vi "查询模块.vi"() -> ()   [LabVIEW 2014]
uses:
  <vilib>/addons/database/Connection.llb/Conn ObjectReference.ctl
  <vilib>/addons/database/NI_Database_API.lvlib
panel:
  in  "返回运行界面":bool
  in  "删除选中数据":bool
  in  "保存为其他格式":bool
  in  "本月":bool
  in  "本周":bool
  in  "今天":bool
  in  "昨天":bool
  in  "查询数据显示表格":i32(listbox)
  in  "error out":errorcluster
  in  "连接输出":T1
  in  "Count":string
  in  "查询输入站号":u16(ring) caption="Station" items=["ALL", "10", "20", "30", "40", "50", "60"]
  in  "查询输入模式":u16(ring) caption="Mode" items=["ALL", "46700-D4100(-P/SW)", "46700-D4200(+P/SW)", "46700-D4300(DCT,-P/SW)", "46700-D4400(DCT,+P/SW)"]
  in  "From":string
  in  "To":string
  out "查询指令":string
  in  "OK":bool
  in  "NG":bool
  in  "ALL":bool
  out "查询界面查询条件":u32
  in  "查询输入S/N":string caption="S/N"
  in  "查询界面查询按钮":bool
  # "46700-D4400(DCT,+P/SW):\n                                       Mode:\n                                                      1:46700-D4100(-P/SW)\n                                                      2:46700-D4200(+P/SW)\n                                                      3:46700-D4300(DCT,-P/SW)\n                                                      4:46700-D4400(DCT,+P/SW)\n1506050001                     :\n                                        150605:YY-MM-DD\n                                        0001    :Count"
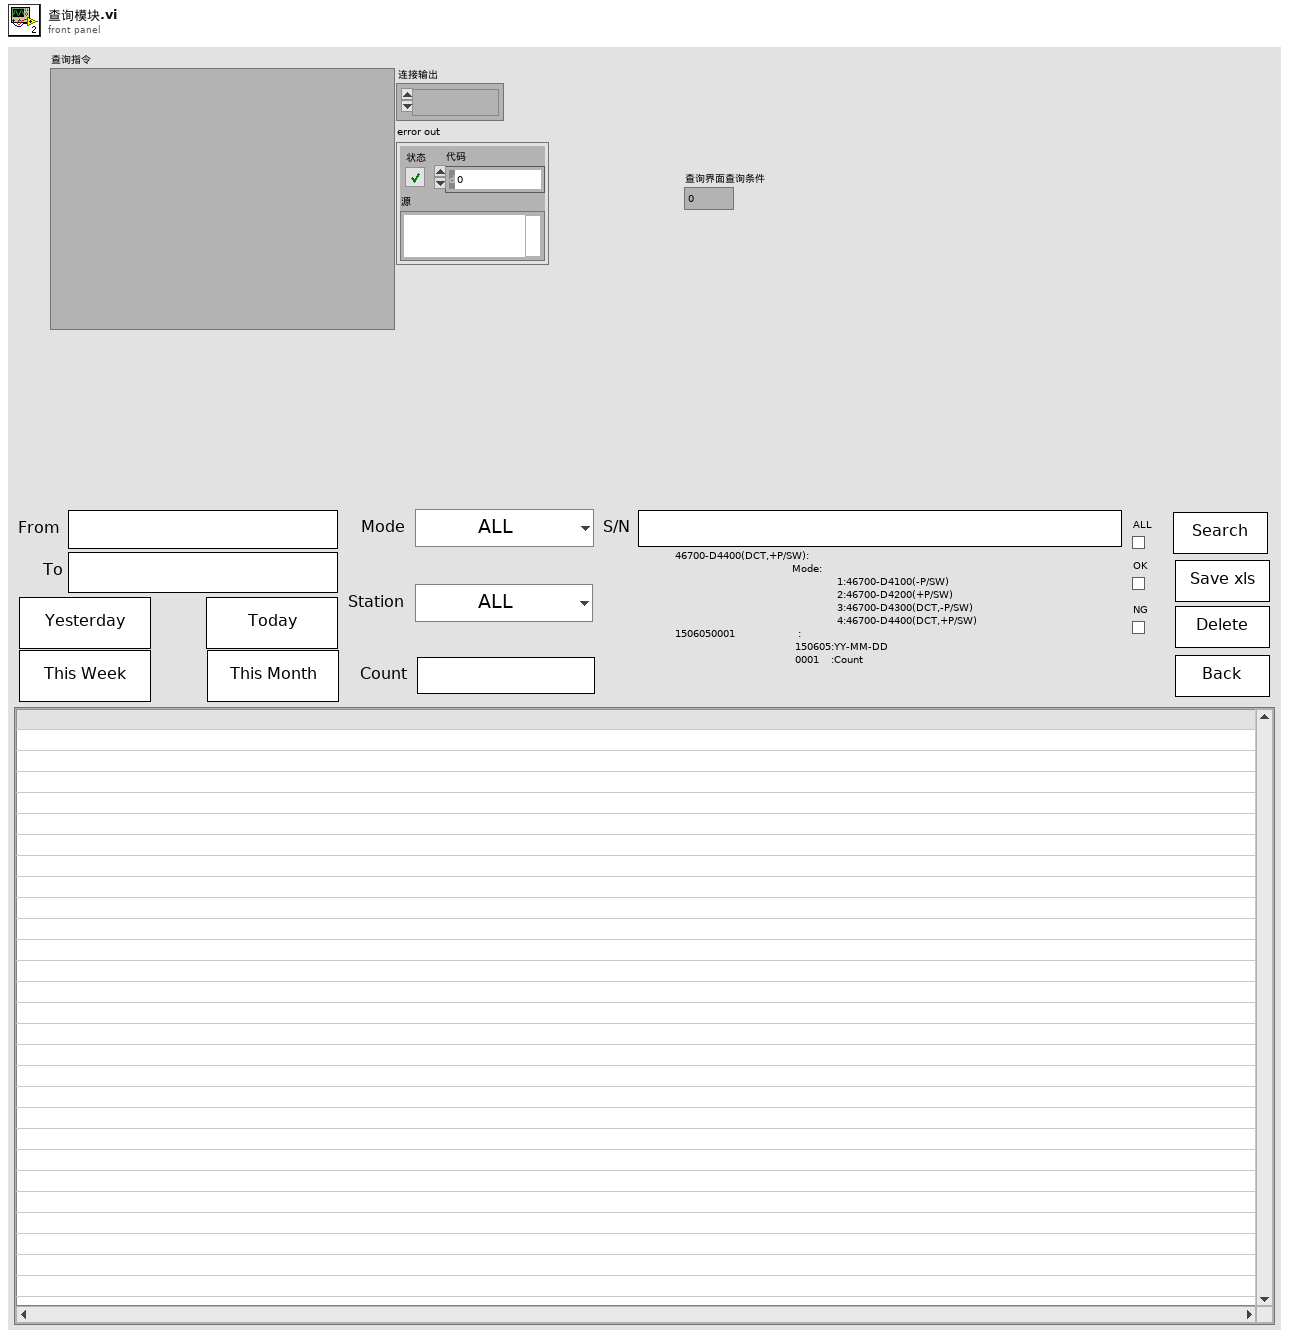
[diagram p1: front panel]
types:
  T1 = typedef "NI_Database_API.lvlib/Conn ObjectReference.ctl" = refnum<k1>
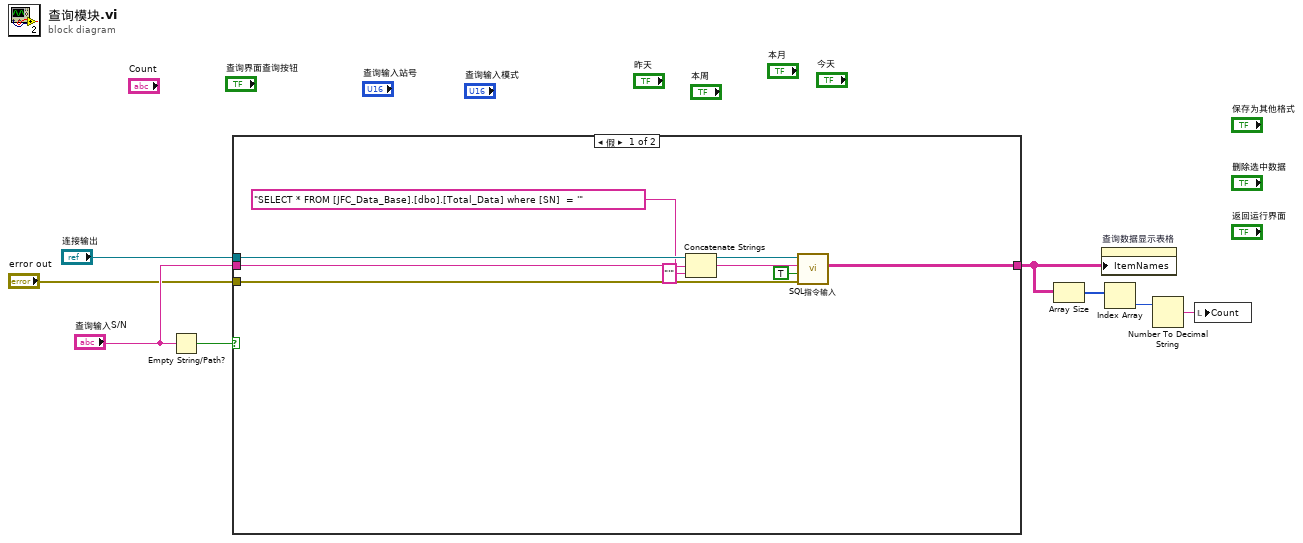
[diagram p0: block diagram]
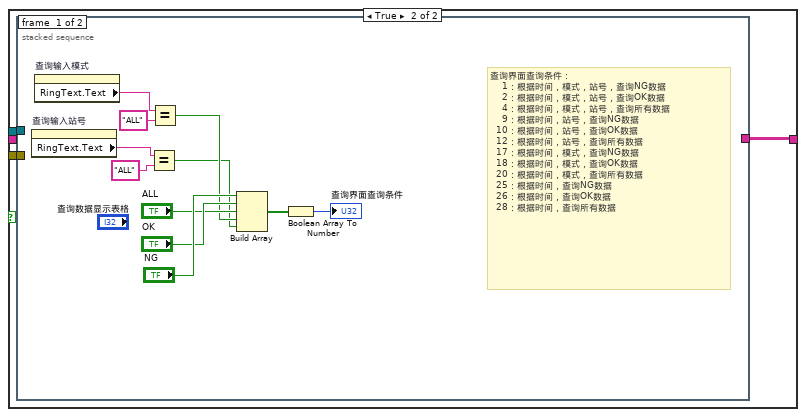
[diagram p2: hidden frame]
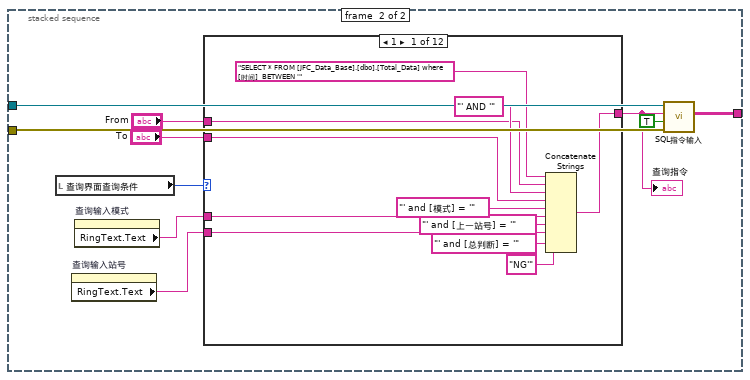
[diagram p3: hidden frame]
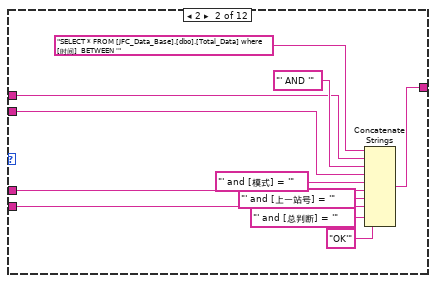
[diagram p4: hidden frame]
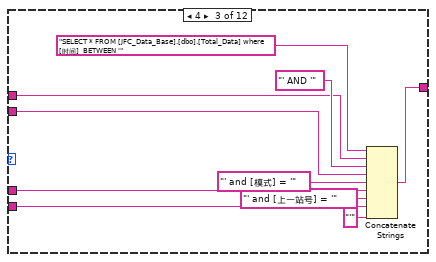
[diagram p5: hidden frame]
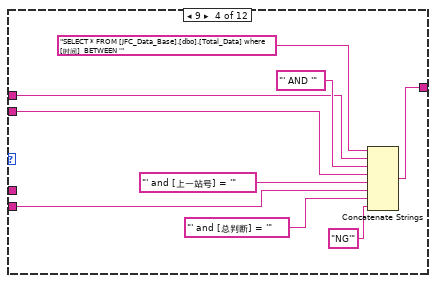
[diagram p6: hidden frame]
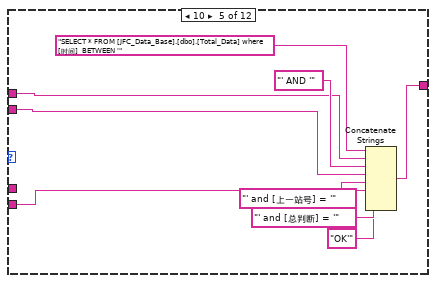
[diagram p7: hidden frame]
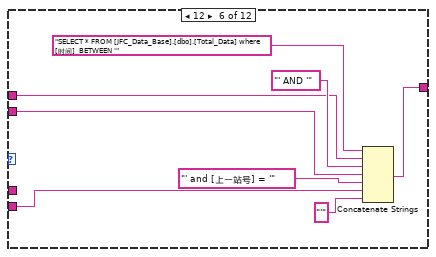
[diagram p8: hidden frame]
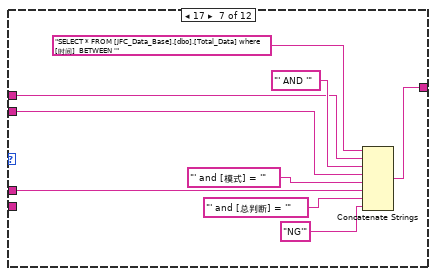
[diagram p9: hidden frame]
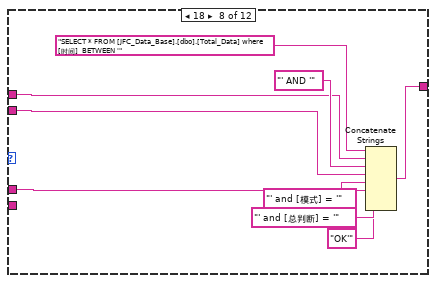
[diagram p10: hidden frame]
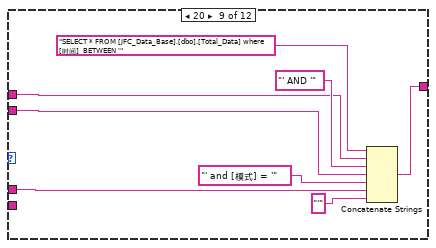
[diagram p11: hidden frame]
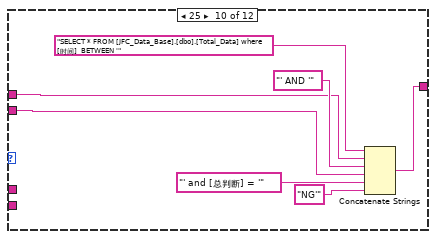
[diagram p12: hidden frame]
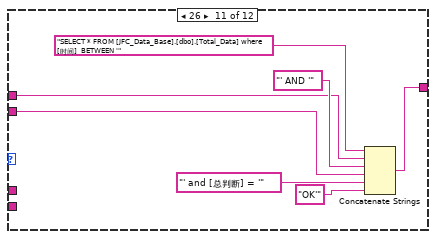
[diagram p13: hidden frame]
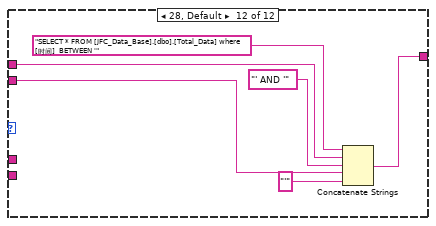
[diagram p14: hidden frame]
diagram:
  n1 = Empty String/Path?(string/path="查询输入S/N") -> (empty?=w8:bool)
  n2 = case shown="假" w8 {
    tunnel: "连接输出" -> [w16 w19]
    tunnel: "error out" -> [w15 w18]
    tunnel: [w13 w17] -> w6
    tunnel: "查询输入S/N" -> [w11 _]
    frame False {
      n3 = Concatenate Strings("SELECT * FROM [JFC_Data_Base].[dbo].[Total_Data] where [SN]  = '" ("SQL query"), w11, "'" ("字符串")) -> (w9:string)
      n4 = call "SQL指令输入.vi"("error in (no error)"=w15, "需要数据？"=TRUE, "SQL query"=w9, "连接输入"=w16) -> ("数据库数据"=w13:string[][])  [unwired: 3 in, 4 out]
    }
    frame True {
      n5 = stacked-sequence {
        tunnel: [_ w40] -> w17
        tunnel: w19 -> [_ w39]
        tunnel: w18 -> [_ w38]
        frame #0 {
          # "查询界面查询条件：\n    1：根据时间，模式，站号，查询NG数据\n    2：根据时间，模式，站号，查询OK数据\n    4：根据时间，模式，站号，查询所有数据\n    9：根据时间，站号，查询NG数据\n  10：根据时间，站号，查询OK数据\n  12：根据时间，站号，查询所有数据\n  17：根据时间，模式，查询NG数据\n  18：根据时间，模式，查询OK数据\n  20：根据时间，模式，查询所有数据\n  25：根据时间，查询NG数据\n  26：根据时间，查询OK数据\n  28：根据时间，查询所有数据"
          n6 = property on="查询输入站号" class="Ring (严格)"() -> ("RingText.Text"=w25:string)  [unwired: 2 in, 2 out]
          n7 = property on="查询输入模式" class="Ring (严格)"() -> ("RingText.Text"=w26:string)  [unwired: 2 in, 2 out]
          n8 = Equal?(x=w25, y="ALL") -> (x = y?=w20:bool)
          n9 = Equal?(x=w26, y="ALL") -> (x = y?=w21:bool)
          n10 = Build Array("NG", "OK", "ALL", w21, w20) -> (w28:bool[])
          n11 = Boolean Array To Number(Boolean array=w28) -> (number=→"查询界面查询条件":u32)
        }
        frame #1 {
          n12 = local read "查询界面查询条件"() -> (w37:u32)
          n13 = property on="查询输入站号" class="Ring (严格)"() -> ("RingText.Text"=w31:string)  [unwired: 2 in, 2 out]
          n14 = property on="查询输入模式" class="Ring (严格)"() -> ("RingText.Text"=w32:string)  [unwired: 2 in, 2 out]
          n15 = case shown="1" w37 {
            tunnel: [w41 w52 w63 w73 w82 w91 w99 w108 w117 w125 w132 w141] -> w36
            tunnel: "From" -> [w49 w56 w67 w76 w85 w95 w102 w111 w120 w127 w134 w140]
            tunnel: "To" -> [w48 w55 w66 w75 w84 w94 w101 w110 w119 w126 w133 w139]
            tunnel: w32 -> [w46 w54 w65 _ _ _ w100 w109 w118 _ _ _]
            tunnel: w31 -> [w44 w53 w64 w74 w83 w93 _ _ _ _ _ _]
            frame 1 {
              n16 = Concatenate Strings("SELECT * FROM [JFC_Data_Base].[dbo].[Total_Data] where [时间]  BETWEEN '" ("SQL query"), w49, "' AND '" ("字符串"), w48, "' and [模式] = '" ("字符串"), w46, "' and [上一站号] = '" ("字符串"), w44, "' and [总判断] = '" ("字符串"), "NG'" ("字符串")) -> (w41:string)
            }
            frame 2 {
              n17 = Concatenate Strings("SELECT * FROM [JFC_Data_Base].[dbo].[Total_Data] where [时间]  BETWEEN '" ("SQL query"), w56, "' AND '" ("字符串"), w55, "' and [模式] = '" ("字符串"), w54, "' and [上一站号] = '" ("字符串"), w53, "' and [总判断] = '" ("字符串"), "OK'" ("字符串")) -> (w52:string)
            }
            frame 4 {
              n18 = Concatenate Strings("SELECT * FROM [JFC_Data_Base].[dbo].[Total_Data] where [时间]  BETWEEN '" ("SQL query"), w67, "' AND '" ("字符串"), w66, "' and [模式] = '" ("字符串"), w65, "' and [上一站号] = '" ("字符串"), w64, "'" ("字符串")) -> (w63:string)
            }
            frame 9 {
              n19 = Concatenate Strings("SELECT * FROM [JFC_Data_Base].[dbo].[Total_Data] where [时间]  BETWEEN '" ("SQL query"), w76, "' AND '" ("字符串"), w75, "' and [上一站号] = '" ("字符串"), w74, "' and [总判断] = '" ("字符串"), "NG'" ("字符串")) -> (w73:string)
            }
            frame 10 {
              n20 = Concatenate Strings("SELECT * FROM [JFC_Data_Base].[dbo].[Total_Data] where [时间]  BETWEEN '" ("SQL query"), w85, "' AND '" ("字符串"), w84, "' and [上一站号] = '" ("字符串"), w83, "' and [总判断] = '" ("字符串"), "OK'" ("字符串")) -> (w82:string)
            }
            frame 12 {
              n21 = Concatenate Strings("SELECT * FROM [JFC_Data_Base].[dbo].[Total_Data] where [时间]  BETWEEN '" ("SQL query"), w95, "' AND '" ("字符串"), w94, "' and [上一站号] = '" ("字符串"), w93, "'" ("字符串")) -> (w91:string)
            }
            frame 17 {
              n22 = Concatenate Strings("SELECT * FROM [JFC_Data_Base].[dbo].[Total_Data] where [时间]  BETWEEN '" ("SQL query"), w102, "' AND '" ("字符串"), w101, "' and [模式] = '" ("字符串"), w100, "' and [总判断] = '" ("字符串"), "NG'" ("字符串")) -> (w99:string)
            }
            frame 18 {
              n23 = Concatenate Strings("SELECT * FROM [JFC_Data_Base].[dbo].[Total_Data] where [时间]  BETWEEN '" ("SQL query"), w111, "' AND '" ("字符串"), w110, "' and [模式] = '" ("字符串"), w109, "' and [总判断] = '" ("字符串"), "OK'" ("字符串")) -> (w108:string)
            }
            frame 20 {
              n24 = Concatenate Strings("SELECT * FROM [JFC_Data_Base].[dbo].[Total_Data] where [时间]  BETWEEN '" ("SQL query"), w120, "' AND '" ("字符串"), w119, "' and [模式] = '" ("字符串"), w118, "'" ("字符串")) -> (w117:string)
            }
            frame 25 {
              n25 = Concatenate Strings("SELECT * FROM [JFC_Data_Base].[dbo].[Total_Data] where [时间]  BETWEEN '" ("SQL query"), w127, "' AND '" ("字符串"), w126, "' and [总判断] = '" ("字符串"), "NG'" ("字符串")) -> (w125:string)
            }
            frame 26 {
              n26 = Concatenate Strings("SELECT * FROM [JFC_Data_Base].[dbo].[Total_Data] where [时间]  BETWEEN '" ("SQL query"), w134, "' AND '" ("字符串"), w133, "' and [总判断] = '" ("字符串"), "OK'" ("字符串")) -> (w132:string)
            }
            frame 28, Default {
              n27 = Concatenate Strings("SELECT * FROM [JFC_Data_Base].[dbo].[Total_Data] where [时间]  BETWEEN '" ("SQL query"), w140, "' AND '" ("字符串"), w139, "'" ("字符串")) -> (w141:string)
            }
          }
          "查询指令" <- w36
          n28 = call "SQL指令输入.vi"("error in (no error)"=w38, "需要数据？"=TRUE, "SQL query"=w36, "连接输入"=w39) -> ("数据库数据"=w40:string[][])  [unwired: 3 in, 4 out]
        }
      }
    }
  }
  n29 = Array Size(array=w6) -> (size(s)=w5:i32[])
  n30 = property on="查询数据显示表格" class="MCListbox (严格)"("ItemNames"=w6) -> ()  [unwired: 2 in, 2 out]
  n31 = Index Array(array=w5) -> (element=w4:i32)  [unwired: 1 in]
  n32 = Number To Decimal String(number=w4) -> (decimal integer string=w3:string)  [unwired: 1 in]
  n33 = local write "Count"(w3) -> ()
